vi "Enqueue Message.vi"(8 "error in (no error)":errorcluster, 9 "Cmd":string, 10 "Data variant":variant, 11 "Queue In":refnum<queue>) -> (0 "error out":errorcluster)   [LabVIEW 2016]
uses:
  Controls/Message Structure.ctl
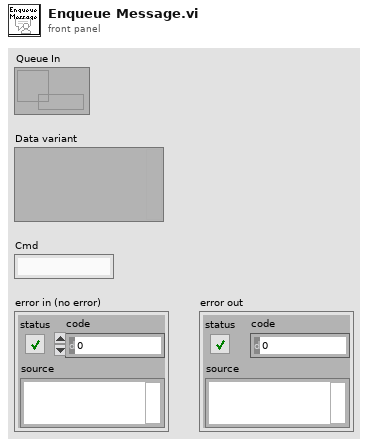
[diagram p1: front panel]
types:
  T1 = typedef "Message Structure.ctl" = cluster{"Data":variant, "Cmd":string}
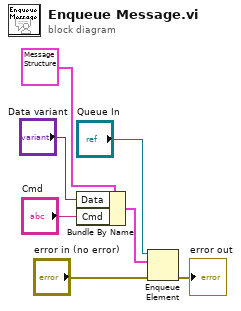
[diagram p0: block diagram]
diagram:
  n1 = Bundle By Name(cluster=T1 {"Data"=variant, "Cmd"=""} ("Message"), "Data"="Data variant", "Cmd"="Cmd") -> (w6:T1)
  n2 = Enqueue Element(queue="Queue In", element=w6, error in (no error)="error in (no error)") -> (error out=→"error out":errorcluster)  [unwired: 1 in, 2 out]
